vi "KH Control.vi"(8 "error in":errorcluster, 11 "Channel Setting":T4=[{"Channel"=enum."Channel 1", "Gain"=enum."1x", "Shunt Resistor"=enum."Open", "Input Config"=enum."SE+ (-gnd)"}, {"Channel"=enum."Channel 2", "Gain"=enum."1x", "Shunt Resistor"=enum."Open", "Input Config"=enum."SE+ (-gnd)"}, {"Channel"=enum."Channel 3", "Gain"=enum."1x", "Shunt Resistor"=enum."Open", "Input Config"=enum."SE+ (-gnd)"}, {"Channel"=enum."Channel 4", "Gain"=enum."1x", "Shunt Resistor"=enum."Open", "Input Config"=enum."SE+ (-gnd)"}, {"Channel"=enum."Channel 5", "Gain"=enum."1x", "Shunt Resistor"=enum."Open", "Input Config"=enum."SE+ (-gnd)"}, {"Channel"=enum."Channel 6", "Gain"=enum."1x", "Shunt Resistor"=enum."Open", "Input Config"=enum."SE+ (-gnd)"}, {"Channel"=enum."Channel 7", "Gain"=enum."1x", "Shunt Resistor"=enum."Open", "Input Config"=enum."SE+ (-gnd)"}, {"Channel"=enum."Channel 8", "Gain"=enum."1x", "Shunt Resistor"=enum."Open", "Input Config"=enum."SE+ (-gnd)"}]) -> (0 "error out":errorcluster={"status"=FALSE, "code"=1073676294, "source"="VISA Read in KH7008 COM.vi->KH7008 Set All.vi->KH Control.vi"})   [LabVIEW 2016]
uses:
  typedefs/KH_control_array.ctl
  typedefs/KH_control.ctl
  typedefs/Channel-Enum.ctl
  typedefs/Gain-Enum.ctl
  typedefs/Shunt-Enum.ctl
  typedefs/Input Configuration-Enum.ctl
  typedefs/SetAll-Cluster.ctl
  typedefs/Filter-Enum.ctl
  typedefs/Coupling-Enum.ctl
  <vilib>/MakerHub/Toolbox/LMH-Toolbox.lvlib
panel:
  in  "All chan same?":bool=TRUE
  in  "Input Configuration":T1=enum."SE+ (-gnd)"
  in  "Shunt Resistor (in diff mode)":T2=enum."50 Ohms"
  in  "Gain":T3
  in  "VISA Refnum in":refnum<visa-resource-name>="COM3"
  # "Measure Current: Current, Shunt Resistor: 50kOhm\nMeasure Voltage: Voltage, Shunt Resistor: Open\nApplying Gate: Current, Shunt Resistor: 50kOhm\n                      Open all the unused gate"
  # "1. Create a copy of drivers under C:\\Krohn-Hite 7008\\Drivers if there is none. \n2. In device manager browse the driver for Krohn-Hite"
  # "Warning: repeated channels will cause false reading in the lock-in"
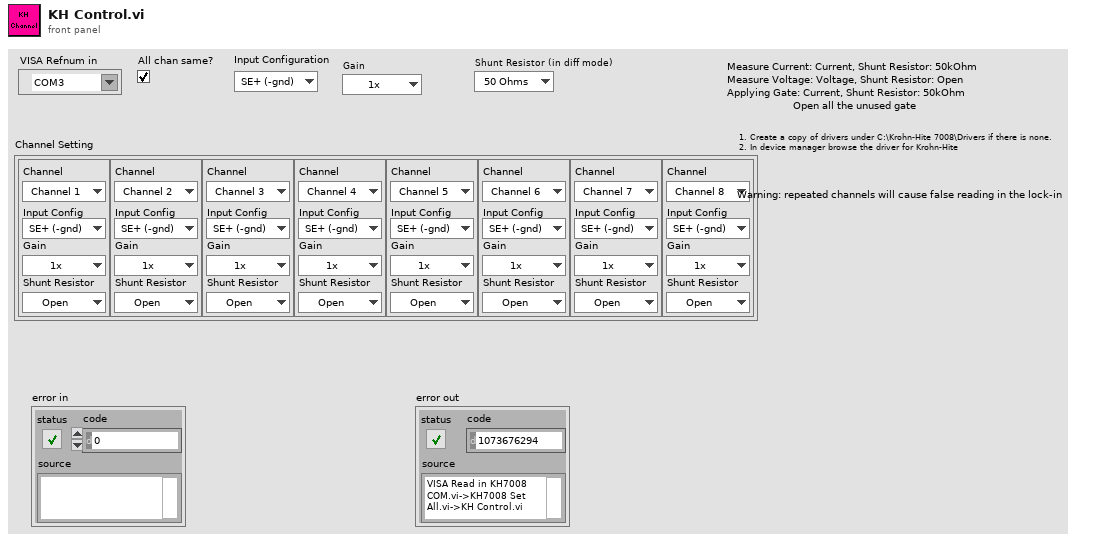
[diagram p1: front panel]
types:
  T1 = typedef "Input Configuration-Enum.ctl" = enum16{"Ground", "SE+ (-gnd)", "SE- (+gnd)", "Differential"}
  T2 = typedef "Shunt-Enum.ctl" = enum16{"Open", "50 Ohms", "500 Ohms", "5k Ohms", "50k Ohms"}
  T3 = typedef "Gain-Enum.ctl" = enum16{"1x", "10x", "100x", "1000x"}
  T4 = typedef "KH_control_array.ctl" = T5[]
  T5 = typedef "KH_control.ctl" = cluster{"Channel":T6, "Gain":T3, "Shunt Resistor":T2, "Input Config":T1}
  T6 = typedef "Channel-Enum.ctl" = enum16{"Channel 1", "Channel 2", "Channel 3", "Channel 4", "Channel 5", "Channel 6", "Channel 7", "Channel 8"}
  T7 = typedef "Coupling-Enum.ctl" = enum16{"AC", "DC"}
  T8 = typedef "Filter-Enum.ctl" = enum16{"OFF", "ON"}
  T9 = typedef "SetAll-Cluster.ctl" = cluster{"Channel":T6, "Gain":T3, "Bandwidth Filter":T8, "Shunt Resistor":T2, "Coupling":T7, "Input Configuration":T1}
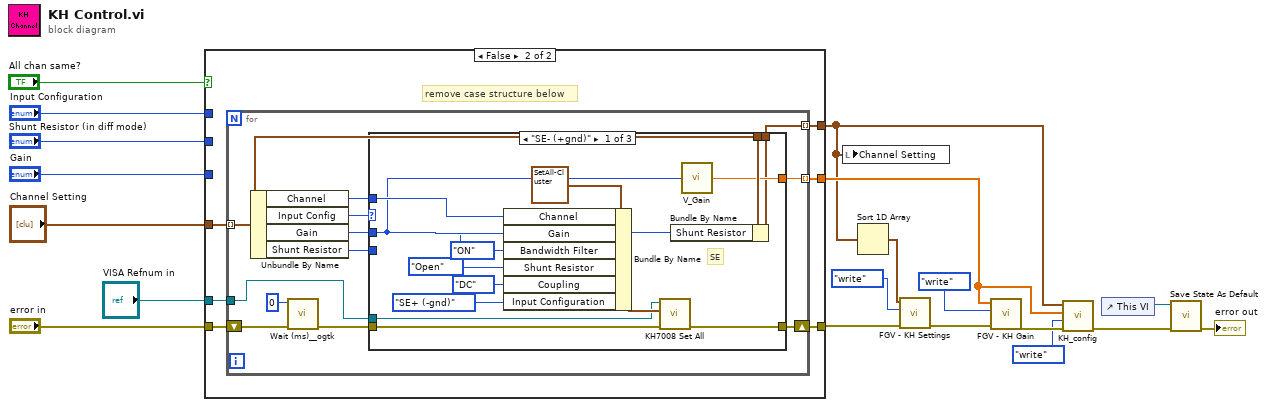
[diagram p0: block diagram]
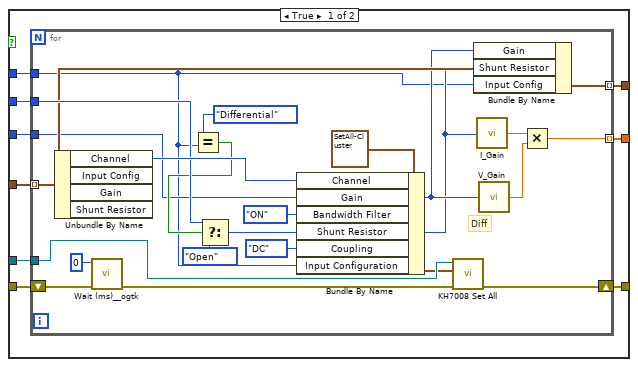
[diagram p2: hidden frame]
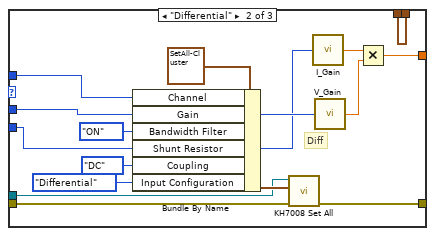
[diagram p3: hidden frame]
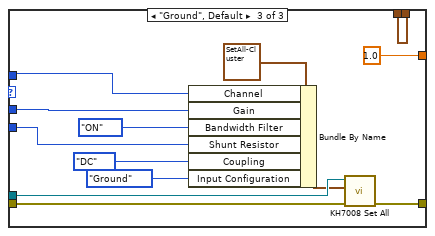
[diagram p4: hidden frame]
diagram:
  n1 = case shown="False" "All chan same?" {
    tunnel: "error in" -> [w28 w56]
    tunnel: [w25 w53] -> w9
    tunnel: [w27 w55] -> w12
    tunnel: "Channel Setting" -> [w26 w54]
    tunnel: [w24 w52] -> w6
    tunnel: "VISA Refnum in" -> [w23 w51]
    tunnel: "Input Configuration" -> [w22 _]
    tunnel: "Shunt Resistor (in diff mode)" -> [w21 _]
    tunnel: "Gain" -> [w20 _]
    frame True {
      n2 = for {
        tunnel: w26 -> [w33] mode=indexing
        tunnel: [w49] -> w27 mode=indexing
        shift-right: [w47] -> w25
        shift-left: w28 -> [w48]
        tunnel: [w32] -> w24 mode=indexing
        tunnel: w23 -> [w44]
        tunnel: w22 -> [w29]
        tunnel: w21 -> [w37]
        tunnel: w20 -> [w31]
        # "Diff"
        n3 = Unbundle By Name(w33) -> ("Channel"=w50:T6)  [unwired: 3 out]
        n4 = call <userlib>:"Wait (ms)__ogtk.vi"("error in (no error)"=w48, "milliseconds to wait"=u32 0) -> ("error out"=w46:errorcluster)  [unwired: 8 in, 1 out]
        n5 = Equal?(x=Input_Configuration-Enum."Differential" ("Input Configuration"), y=w29) -> (x = y?=w34:bool)
        n6 = Select(t=w37, s=w34, f=Shunt-Enum."Open") -> (s? t:f=w30:T2)
        n7 = Bundle By Name(cluster=T9 {"Channel"=enum."Channel 2", "Gain"=enum."10x", "Bandwidth Filter"=enum."ON", "Shunt Resistor"=enum."50 Ohms", "Coupling"=enum."DC", "Input Configuration"=enum."Differential"} ("Set All"), "Channel"=w50, "Gain"=w31, "Bandwidth Filter"=Filter-Enum."ON", "Shunt Resistor"=w30, "Coupling"=Coupling-Enum."DC", "Input Configuration"=w29) -> (w40:T9)
        n8 = call "KH7008 Set All.vi"("error in (no error)"=w46, "Set All"=w40, "VISA Refnum in"=w44) -> ("error out"=w47:errorcluster)  [unwired: 4 in]
        n9 = Bundle By Name(cluster=w33, "Gain"=w31, "Shunt Resistor"=w30, "Input Config"=w29) -> (w32:T5)
        n10 = call "I_Gain.vi"("Shunt Resistor"=w30) -> ("Gain (V/A)"=w39:dbl)
        n11 = call "V_Gain.vi"("Gain"=w31) -> ("Gain (x)"=w38:dbl)
        n12 = Multiply(x=w39, y=w38) -> (x*y=w49:dbl)
      }
    }
    frame False {
      # "remove case structure below"
      n13 = for {
        tunnel: w54 -> [w59] mode=indexing
        tunnel: [w64] -> w55 mode=indexing
        shift-right: [w62] -> w53
        shift-left: w56 -> [w63]
        tunnel: [w58] -> w52 mode=indexing
        tunnel: w51 -> [w57]
        n14 = Unbundle By Name(w59) -> ("Channel"=w68:T6, "Input Config"=w65:T1, "Gain"=w67:T3, "Shunt Resistor"=w66:T2)
        n15 = call <userlib>:"Wait (ms)__ogtk.vi"("error in (no error)"=w63, "milliseconds to wait"=u32 0) -> ("error out"=w61:errorcluster)  [unwired: 8 in, 1 out]
        n16 = case shown="\"SE- (+gnd)\"" w65 {
          tunnel: w68 -> [w77 w93 w105]
          tunnel: w67 -> [w73 w86 w104]
          tunnel: w66 -> [_ w84 w102]
          tunnel: w57 -> [w78 w88 w108]
          tunnel: [w72 w97 1.0] -> w64
          tunnel: w61 -> [w80 w95 w110]
          tunnel: [w81 w94 w109] -> w62
          tunnel: w59 -> [w74 w83 w98]
          tunnel: [w71 w83 w98] -> w58
          frame "SE- (+gnd)" {
            w70 = Shunt-Enum."Open" ("Shunt Resistor")
            # "SE"
            n17 = Bundle By Name(cluster=T9 {"Channel"=enum."Channel 2", "Gain"=enum."10x", "Bandwidth Filter"=enum."ON", "Shunt Resistor"=enum."50 Ohms", "Coupling"=enum."DC", "Input Configuration"=enum."Differential"} ("Set All"), "Channel"=w77, "Gain"=w73, "Bandwidth Filter"=Filter-Enum."ON", "Shunt Resistor"=w70, "Coupling"=Coupling-Enum."DC", "Input Configuration"=Input_Configuration-Enum."SE+ (-gnd)") -> (w79:T9)
            n18 = call "KH7008 Set All.vi"("error in (no error)"=w80, "Set All"=w79, "VISA Refnum in"=w78) -> ("error out"=w81:errorcluster)  [unwired: 4 in]
            n19 = Bundle By Name(cluster=w74, "Shunt Resistor"=w70) -> (w71:T5)
            n20 = call "V_Gain.vi"("Gain"=w73) -> ("Gain (x)"=w72:dbl)
          }
          frame "Differential" {
            # "Diff"
            n21 = Bundle By Name(cluster=T9 {"Channel"=enum."Channel 2", "Gain"=enum."10x", "Bandwidth Filter"=enum."ON", "Shunt Resistor"=enum."50 Ohms", "Coupling"=enum."DC", "Input Configuration"=enum."Differential"} ("Set All"), "Channel"=w93, "Gain"=w86, "Bandwidth Filter"=Filter-Enum."ON", "Shunt Resistor"=w84, "Coupling"=Coupling-Enum."DC", "Input Configuration"=Input_Configuration-Enum."Differential") -> (w89:T9)
            n22 = call "KH7008 Set All.vi"("error in (no error)"=w95, "Set All"=w89, "VISA Refnum in"=w88) -> ("error out"=w94:errorcluster)  [unwired: 4 in]
            n23 = call "I_Gain.vi"("Shunt Resistor"=w84) -> ("Gain (V/A)"=w87:dbl)
            n24 = call "V_Gain.vi"("Gain"=w86) -> ("Gain (x)"=w85:dbl)
            n25 = Multiply(x=w87, y=w85) -> (x*y=w97:dbl)
          }
          frame "Ground", Default {
            n26 = Bundle By Name(cluster=T9 {"Channel"=enum."Channel 2", "Gain"=enum."10x", "Bandwidth Filter"=enum."ON", "Shunt Resistor"=enum."50 Ohms", "Coupling"=enum."DC", "Input Configuration"=enum."Differential"} ("Set All"), "Channel"=w105, "Gain"=w104, "Bandwidth Filter"=Filter-Enum."ON", "Shunt Resistor"=w102, "Coupling"=Coupling-Enum."DC", "Input Configuration"=Input_Configuration-Enum."Ground") -> (w106:T9)
            n27 = call "KH7008 Set All.vi"("error in (no error)"=w110, "Set All"=w106, "VISA Refnum in"=w108) -> ("error out"=w109:errorcluster)  [unwired: 4 in]
          }
        }
      }
    }
  }
  n28 = local write "Channel Setting"(w6) -> ()
  n29 = Sort 1D Array(array=w6) -> (sorted array=w7:T5[])
  n30 = call "FGV - KH Settings.vi"("error in"=w9, "Function"=enum16{"write", "read"}."write", "Channel Setting"=w7) -> ("error out"=w10:errorcluster)  [unwired: 3 in, 1 out]
  n31 = call "FGV - KH Gain.vi"("error in"=w10, "Function"=enum16{"write", "read"}."write", "Gains"=w12) -> ("error out"=w14:errorcluster)  [unwired: 3 in, 1 out]
  n32 = call "KH_config.vi"("Error In"=w14, "Function"=enum16{"write", "read"}."write", "Gains"=w12, "Channel Setting"=w6) -> ("Error Out"=w15:errorcluster)  [unwired: 5 in, 2 out]
  n33 = control-ref of="This VI"() -> (w18:refnum<vi>)
  n34 = call <vilib>:"Save State As Default.vi"("Error In"=w15, "Target VI"=w18) -> ("Error Out"=→"error out":errorcluster)  [unwired: 8 in, 1 out]
